vi "Buffer Underflow.vi"(7 "error source vi name":string, 8 "error in (no error)":errorcluster, 9 "actual buffer size":u64 format="%d bytes", 10 "required buffer size":u64 format="%d bytes", 11 "Pointer in":refnum<class "Pointer.lvclass">) -> (0 "error out":errorcluster, 3 "Pointer out":refnum<class "Pointer.lvclass">)   [LabVIEW 2017, in "Memory Manager.lvlib" / "Pointer.lvclass"]
uses:
  Pointer.lvclass
  Errors.ctl
  VIs/Write Numeric Scalar to Source (Base10 U64).vi
  Static Errors.lvlib
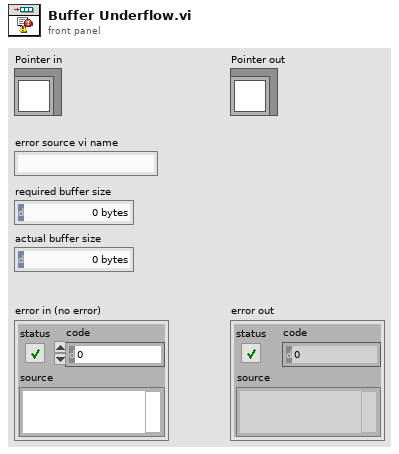
[diagram p1: front panel]
types:
  T1 = typedef "Memory Manager.lvlib/Pointer.lvclass/Errors.ctl" = enum16{"No Error", "Null Pointer", "Out of Bounds", "Buffer Underflow", "Size Mismatch", "Zone"}
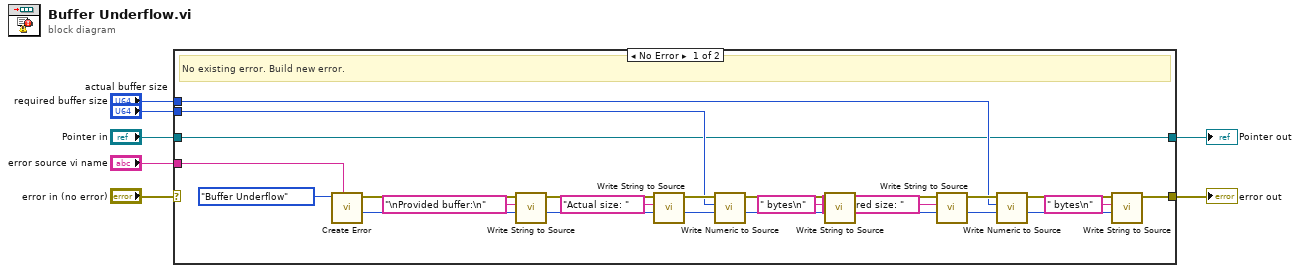
[diagram p0: block diagram]
diagram:
  n1 = case shown="No Error" "error in (no error)" {
    selector: "error in (no error)" -> [_ w34]
    tunnel: [w15 w34] -> w4
    tunnel: "actual buffer size" -> [w27 _]
    tunnel: "error source vi name" -> [w31 _]
    tunnel: "Pointer in" -> [w10 w33]
    tunnel: [w10 w33] -> w2
    tunnel: "required buffer size" -> [w14 _]
    frame No Error {
      # "No existing error. Build new error."
      n2 = call "Create Error.vi"("source vi name"=w31, "error"=Errors."Buffer Underflow") -> ("new offset"=w8:i32, "error out"=w9:errorcluster)  [unwired: 8 in]
      n3 = call "Write String to Source.vi"("offset"=w8, "string"="\nProvided buffer:\n", "error in"=w9) -> ("new offset"=w12:i32, "error out"=w13:errorcluster)  [unwired: 7 in]
      n4 = call "Write String to Source.vi"("offset"=w12, "string"="Actual size: ", "error in"=w13) -> ("new offset"=w28:i32, "error out"=w29:errorcluster)  [unwired: 7 in]
      n5 = call-poly "Write Numeric to Source.vi"("offset"=w28, "value"=w27, "error in"=w29) -> ("new offset"=w24:i32, "error out"=w25:errorcluster)  [unwired: 7 in]
      n6 = call "Write String to Source.vi"("offset"=w24, "string"=" bytes\n", "error in"=w25) -> ("new offset"=w16:i32, "error out"=w17:errorcluster)  [unwired: 7 in]
      n7 = call "Write String to Source.vi"("offset"=w16, "string"="Required size: ", "error in"=w17) -> ("new offset"=w21:i32, "error out"=w22:errorcluster)  [unwired: 7 in]
      n8 = call-poly "Write Numeric to Source.vi"("offset"=w21, "value"=w14, "error in"=w22) -> ("new offset"=w18:i32, "error out"=w19:errorcluster)  [unwired: 7 in]
      n9 = call "Write String to Source.vi"("offset"=w18, "string"=" bytes\n", "error in"=w19) -> ("error out"=w15:errorcluster)  [unwired: 7 in, 1 out]
    }
    frame Error {
      # "Incoming error. Pass through."
    }
  }
  "error out" <- w4
  "Pointer out" <- w2
